vi "LoadAdvancedSettings.vi"(2 "Software settings in":T2, 3 "Hardware settings in":T3, 4 "OCT in":T1) -> (0 "Software settings out":T2, 1 "Hardware  settings out":T3)   [LabVIEW 2017]
uses:
  classes/HardwareObjects/Spectrometer/Spectrometer.lvclass
  classes/HardwareObjects/Camera/Camera.lvclass
  classes/HardwareObjects/DAQ/DAQ.lvclass
  classes/HardwareObjects/Galvonometer/Galvonometer.lvclass
  classes/HardwareObjects/PC/PC.lvclass
  classes/SoftwareObjects/ConfigProc/ConfigProc.lvclass
  classes/HardwareObjects/Galvonometer/Galvonometer.lvclass/Galvonometer.ctl
  classes/SoftwareObjects/ConfigProc/ConfigProc.lvclass/ConfigProc.ctl
  classes/HardwareObjects/Spectrometer/Spectrometer.lvclass/Spectrometer.ctl
  classes/HardwareObjects/DAQ/DAQ.lvclass/DAQ.ctl
  classes/HardwareObjects/PC/PC.lvclass/PC.ctl
  classes/HardwareObjects/Camera/Camera.lvclass/Camera.ctl
  classes/HardwareObjects/Camera/Read Bit Depth.vi
  classes/HardwareObjects/Camera/Read Duty Cycle.vi
  classes/HardwareObjects/Camera/Read Data Representation.vi
  classes/HardwareObjects/Camera/Read Max Frequency (kHz).vi
  classes/HardwareObjects/Camera/Read Return Time (us).vi
  classes/HardwareObjects/Camera/Read Make, Model.vi
  classes/HardwareObjects/Camera/Read Camera Dimensions.vi
  classes/HardwareObjects/PC/Read Max Number of Cores.vi
  classes/HardwareObjects/PC/Read Path to DLL.vi
  classes/HardwareObjects/DAQ/Read Camera Counter.vi
  classes/HardwareObjects/DAQ/Read Camera Counter Output Terminal.vi
  classes/HardwareObjects/DAQ/Read Galvo Counter.vi
  classes/HardwareObjects/DAQ/Read Galvo Counter Terminal.vi
  classes/HardwareObjects/DAQ/Read Master Counter.vi
  classes/HardwareObjects/DAQ/Read Master Counter Terminal.vi
  classes/HardwareObjects/DAQ/Read Galvo Analog Output Channel(s).vi
  classes/HardwareObjects/Spectrometer/Read Bandwidth (nm).vi
  classes/HardwareObjects/Spectrometer/Read Center wavelength (nm).vi
  classes/HardwareObjects/Spectrometer/Read Make Model.vi
  classes/HardwareObjects/Spectrometer/Read Scan depth (mm).vi
  classes/SoftwareObjects/ConfigProc/Read Blur Coefficient.vi
  classes/SoftwareObjects/ConfigProc/Read Blur Int.vi
  classes/SoftwareObjects/ConfigProc/Read Cores.vi
  classes/SoftwareObjects/ConfigProc/Read Interpolation.vi
  classes/SoftwareObjects/ConfigProc/Read Magnification.vi
  classes/SoftwareObjects/ConfigProc/Read Power.vi
  classes/SoftwareObjects/ConfigProc/Read Soften.vi
  classes/SoftwareObjects/ConfigProc/Read Weight.vi
  classes/HardwareObjects/Galvonometer/Read Make Model.vi
  classes/HardwareObjects/Galvonometer/Read Max Scan Angle (degrees).vi
  classes/HardwareObjects/Galvonometer/Read Output Scale Factor (V_degrees).vi
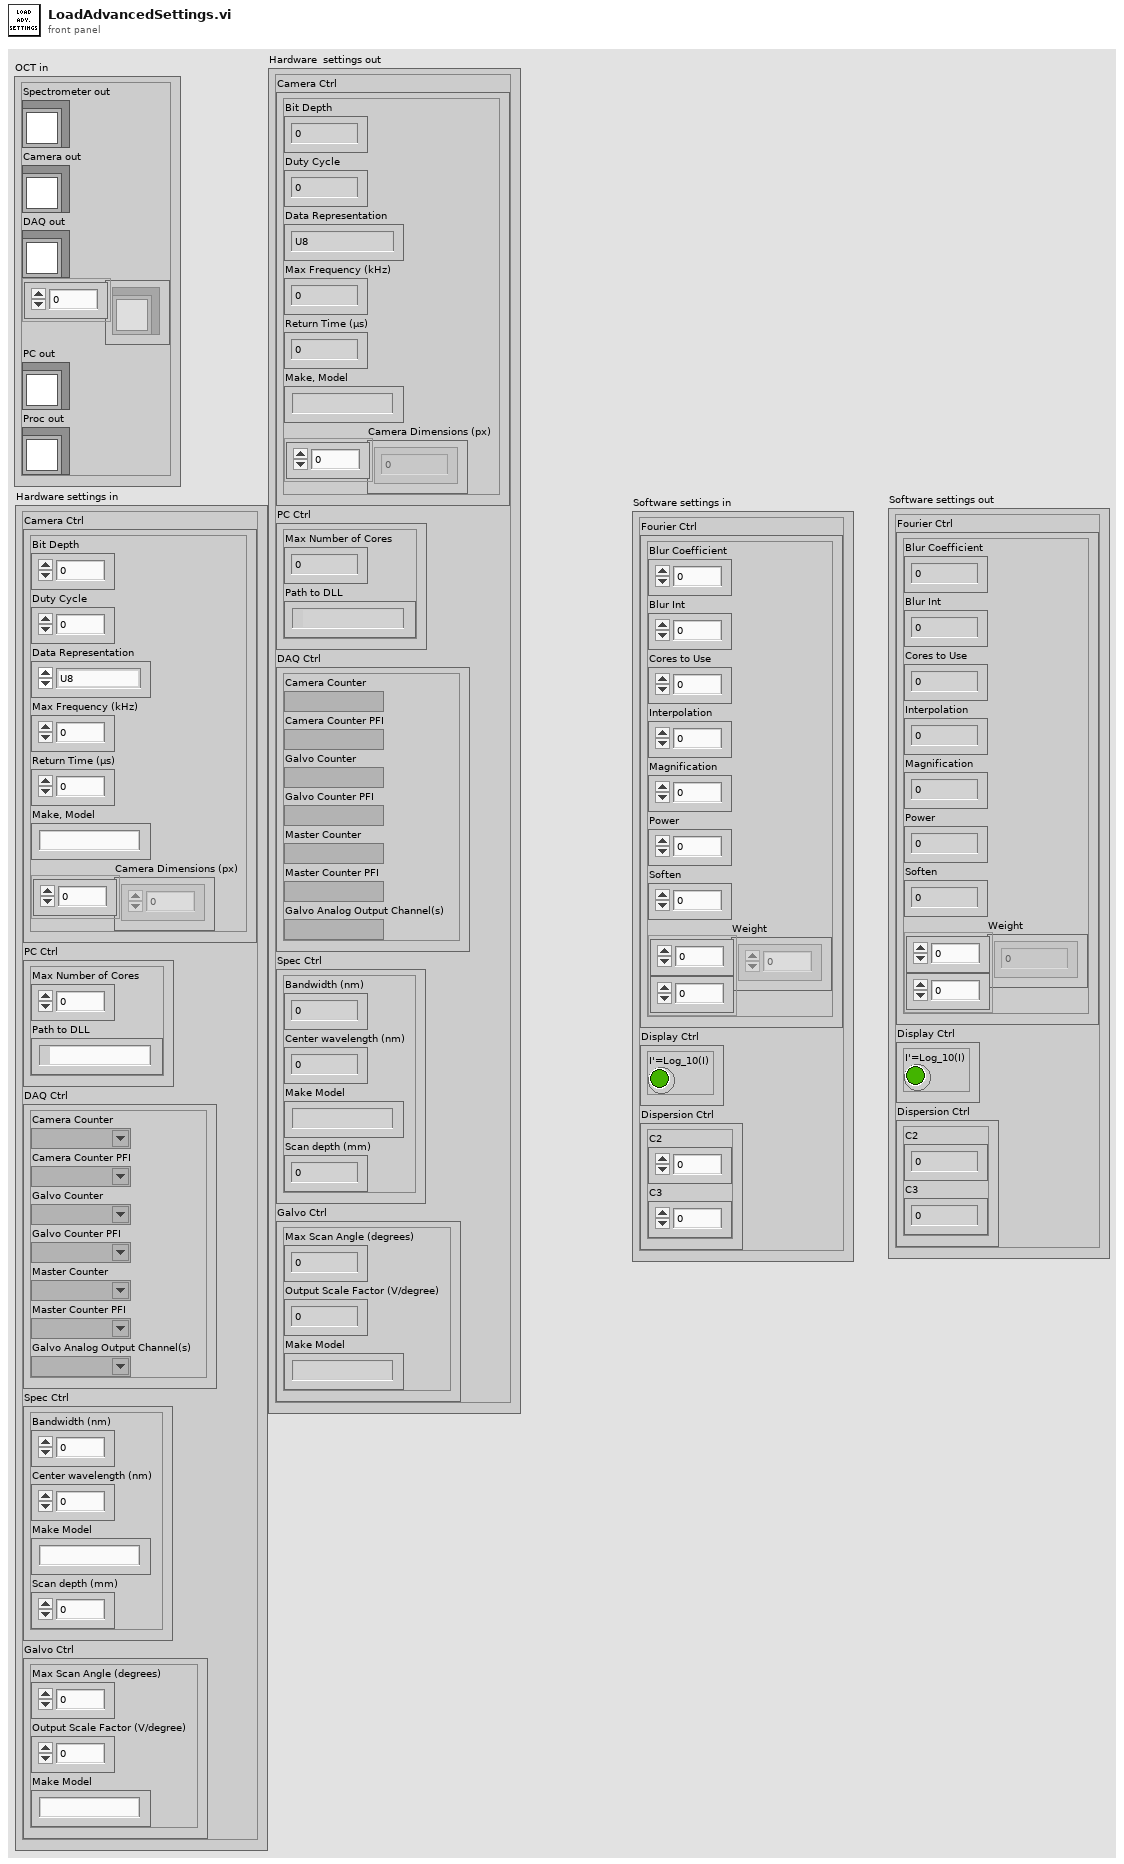
[diagram p1: front panel]
types:
  T1 = cluster{"Spectrometer out":refnum<class "Spectrometer.lvclass">, "Camera out":refnum<class "Camera.lvclass">, "DAQ out":refnum<class "DAQ.lvclass">, "Array":refnum<class "Galvonometer.lvclass">[], "PC out":refnum<class "PC.lvclass">, "Proc out":refnum<class "ConfigProc.lvclass">}
  T2 = cluster{"Fourier Ctrl":cluster{"Blur Coefficient":dbl, "Blur Int":dbl, "Cores to Use":dbl, "Interpolation":dbl, "Magnification":dbl, "Power":dbl, "Soften":dbl, "Weight":cdb[][]}, "Display Ctrl":cluster{"I'=Log_10(I)":bool}, "Dispersion Ctrl":cluster{"C2":dbl, "C3":dbl}}
  T3 = cluster{"Camera Ctrl":cluster{"Bit Depth":dbl, "Duty Cycle":sgl, "Data Representation":enum16{"U8", "I8", "U16", "I16"}, "Max Frequency (kHz)":sgl, "Return Time (µs)":sgl, "Make, Model":string, "Camera Dimensions (px)":u16[]}, "PC Ctrl":cluster{"Max Number of Cores":dbl, "Path to DLL":path}, "DAQ Ctrl":cluster{"Camera Counter":tag, "Camera Counter PFI":tag, "Galvo Counter":tag, "Galvo Counter PFI":tag, "Master Counter":tag, "Master Counter PFI":tag, "Galvo Analog Output Channel(s)":tag}, "Spec Ctrl":cluster{"Bandwidth (nm)":dbl, "Center wavelength (nm)":dbl, "Make Model":string, "Scan depth (mm)":dbl}, "Galvo Ctrl":cluster{"Max Scan Angle (degrees)":dbl, "Output Scale Factor (V/degree)":dbl, "Make Model":string}}
  T4 = cluster{"Blur Coefficient":dbl, "Blur Int":dbl, "Cores to Use":dbl, "Interpolation":dbl, "Magnification":dbl, "Power":dbl, "Soften":dbl, "Weight":cdb[][]}
  T5 = cluster{"Bit Depth":dbl, "Duty Cycle":sgl, "Data Representation":enum16{"U8", "I8", "U16", "I16"}, "Max Frequency (kHz)":sgl, "Return Time (µs)":sgl, "Make, Model":string, "Camera Dimensions (px)":u16[]}
  T6 = cluster{"Max Number of Cores":dbl, "Path to DLL":path}
  T7 = cluster{"Camera Counter":tag, "Camera Counter PFI":tag, "Galvo Counter":tag, "Galvo Counter PFI":tag, "Master Counter":tag, "Master Counter PFI":tag, "Galvo Analog Output Channel(s)":tag}
  T8 = cluster{"Max Scan Angle (degrees)":dbl, "Output Scale Factor (V/degree)":dbl, "Make Model":string}
  T9 = cluster{"Bandwidth (nm)":dbl, "Center wavelength (nm)":dbl, "Make Model":string, "Scan depth (mm)":dbl}
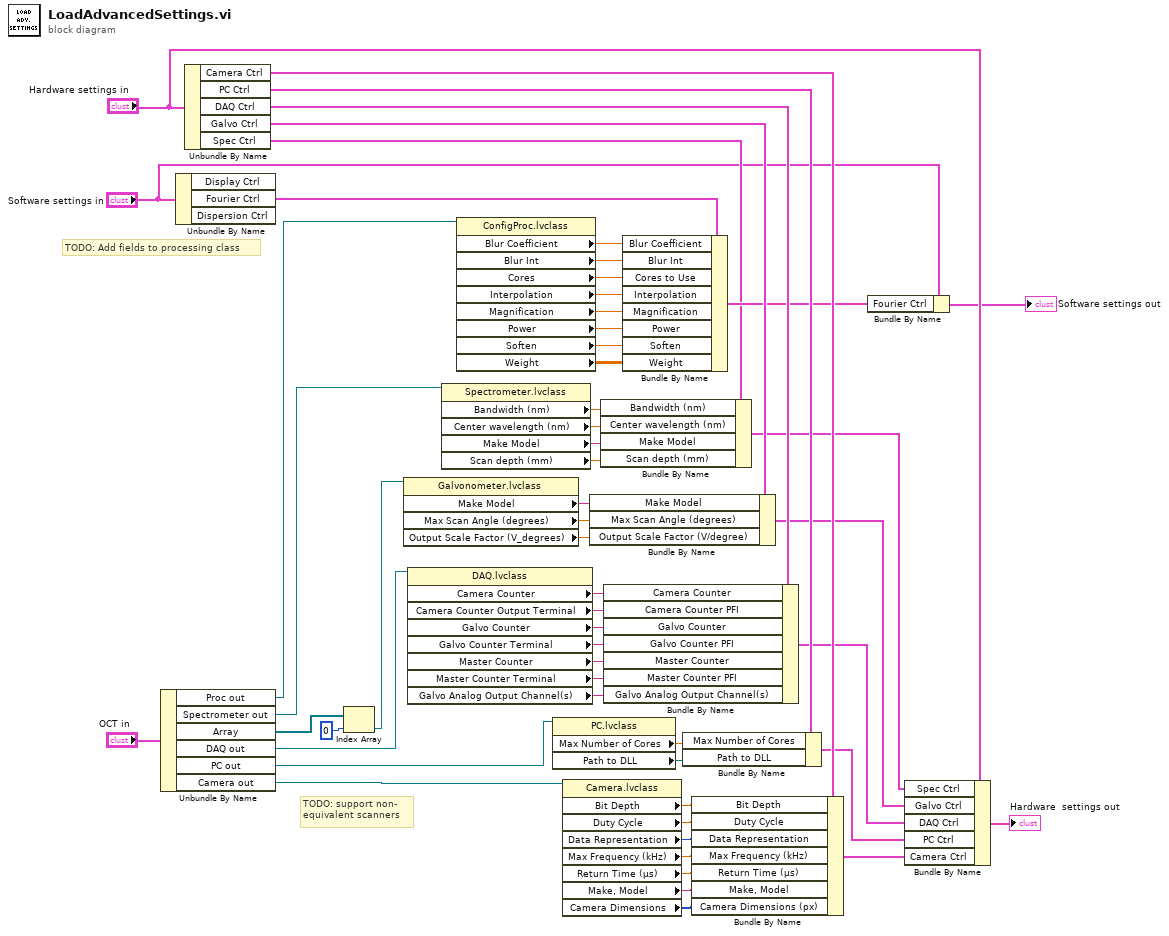
[diagram p0: block diagram]
diagram:
  # "TODO: Add fields to processing class"
  # "TODO: support non-\nequivalent scanners"
  n1 = Unbundle By Name("OCT in") -> ("Proc out"=w12:refnum<class "ConfigProc.lvclass">, "Spectrometer out"=w10:refnum<class "Spectrometer.lvclass">, "Array"=w29:refnum<class "Galvonometer.lvclass">[], "DAQ out"=w42:refnum<class "DAQ.lvclass">, "PC out"=w43:refnum<class "PC.lvclass">, "Camera out"=w54:refnum<class "Camera.lvclass">)
  n2 = Unbundle By Name("Software settings in") -> ("Fourier Ctrl"=w21:T4)  [unwired: 2 out]
  n3 = Unbundle By Name("Hardware settings in") -> ("Camera Ctrl"=w56:T5, "PC Ctrl"=w46:T6, "DAQ Ctrl"=w40:T7, "Galvo Ctrl"=w26:T8, "Spec Ctrl"=w9:T9)
  n4 = Index Array(array=w29, index=0) -> (element=w27:refnum<class "Galvonometer.lvclass">)
  n5 = property class="Galvonometer.lvclass"(reference=w27) -> ("Make Model"=w23:string, "Max Scan Angle (degrees)"=w24:dbl, "Output Scale Factor (V_degrees)"=w25:dbl)  [unwired: 1 in, 2 out]
  n6 = property class="DAQ.lvclass"(reference=w42) -> ("Camera Counter"=w34:tag, "Camera Counter Output Terminal"=w35:tag, "Galvo Counter"=w36:tag, "Galvo Counter Terminal"=w37:tag, "Master Counter"=w38:tag, "Master Counter Terminal"=w39:tag, "Galvo Analog Output Channel(s)"=w31:tag)  [unwired: 1 in, 2 out]
  n7 = property class="Spectrometer.lvclass"(reference=w10) -> ("Bandwidth (nm)"=w5:dbl, "Center wavelength (nm)"=w6:dbl, "Make Model"=w7:string, "Scan depth (mm)"=w8:dbl)  [unwired: 1 in, 2 out]
  n8 = property class="ConfigProc.lvclass"(reference=w12) -> ("Blur Coefficient"=w20:dbl, "Blur Int"=w19:dbl, "Cores"=w18:dbl, "Interpolation"=w17:dbl, "Magnification"=w16:dbl, "Power"=w15:dbl, "Soften"=w14:dbl, "Weight"=w13:cdb[][])  [unwired: 1 in, 2 out]
  n9 = property class="PC.lvclass"(reference=w43) -> ("Max Number of Cores"=w45:dbl, "Path to DLL"=w44:path)  [unwired: 1 in, 2 out]
  n10 = property class="Camera.lvclass"(reference=w54) -> ("Bit Depth"=w47:dbl, "Duty Cycle"=w48:sgl, "Data Representation"=w49:enum16{"U8", "I8", "U16", "I16"}, "Max Frequency (kHz)"=w50:sgl, "Return Time (µs)"=w51:sgl, "Make, Model"=w52:string, "Camera Dimensions"=w53:u16[])  [unwired: 1 in, 2 out]
  n11 = Bundle By Name(cluster=w26, "Make Model"=w23, "Max Scan Angle (degrees)"=w24, "Output Scale Factor (V/degree)"=w25) -> (w22:T8)
  n12 = Bundle By Name(cluster=w9, "Bandwidth (nm)"=w5, "Center wavelength (nm)"=w6, "Make Model"=w7, "Scan depth (mm)"=w8) -> (w4:T9)
  n13 = Bundle By Name(cluster=w40, "Camera Counter"=w34, "Camera Counter PFI"=w35, "Galvo Counter"=w36, "Galvo Counter PFI"=w37, "Master Counter"=w38, "Master Counter PFI"=w39, "Galvo Analog Output Channel(s)"=w31) -> (w33:T7)
  n14 = Bundle By Name(cluster=w21, "Blur Coefficient"=w20, "Blur Int"=w19, "Cores to Use"=w18, "Interpolation"=w17, "Magnification"=w16, "Power"=w15, "Soften"=w14, "Weight"=w13) -> (w11:T4)
  n15 = Bundle By Name(cluster=w46, "Max Number of Cores"=w45, "Path to DLL"=w44) -> (w41:T6)
  n16 = Bundle By Name(cluster=w56, "Bit Depth"=w47, "Duty Cycle"=w48, "Data Representation"=w49, "Max Frequency (kHz)"=w50, "Return Time (µs)"=w51, "Make, Model"=w52, "Camera Dimensions (px)"=w53) -> (w55:T5)
  n17 = Bundle By Name(cluster="Software settings in", "Fourier Ctrl"=w11) -> (→"Software settings out":T2)
  n18 = Bundle By Name(cluster="Hardware settings in", "Spec Ctrl"=w4, "Galvo Ctrl"=w22, "DAQ Ctrl"=w33, "PC Ctrl"=w41, "Camera Ctrl"=w55) -> (→"Hardware  settings out":T3)
